vi "Ordena_Tags.vi"(0 "Tags_desorden":string[](array[string])) -> (1 "sorted array":i32[](array[numeric]), 2 "Array":string[](array[string]))   [LabVIEW 2015]
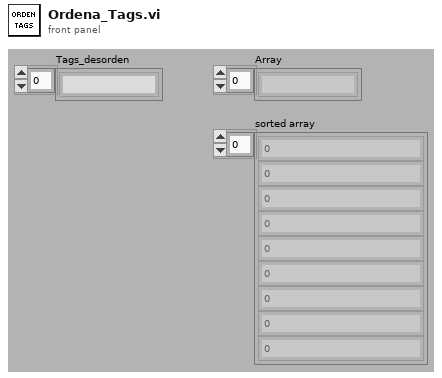
[diagram p1: front panel]
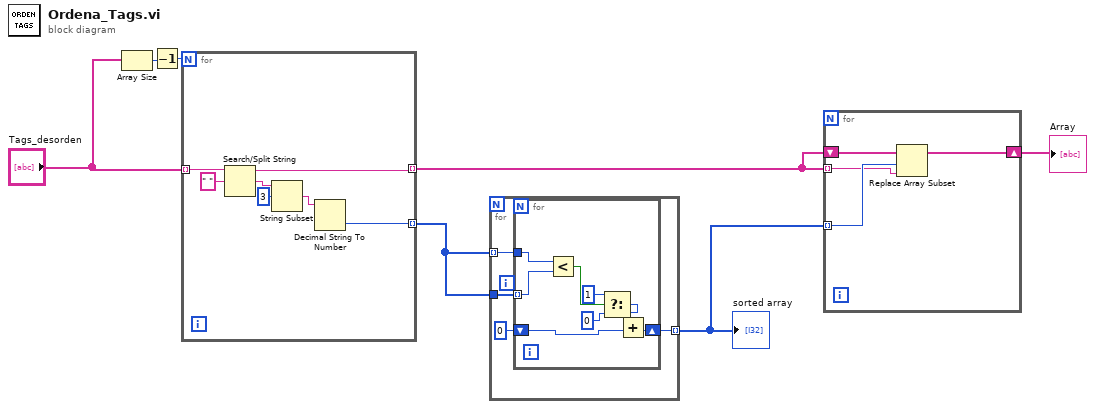
[diagram p0: block diagram]
diagram:
  n1 = Array Size(array="Tags_desorden") -> (size(s)=w1:i32)
  n2 = Decrement(x=w1) -> (x-1=w2:i32)
  n3 = for {
    N: w2 -> [_]
    tunnel: "Tags_desorden" -> [w14] mode=indexing
    tunnel: [w12] -> w5 mode=indexing
    tunnel: [w8] -> w3 mode=indexing
    n4 = Search/Split String(string=w14, search string/char (-)=" ") -> (substring before match=w12:string, match + rest of string=w11:string)  [unwired: 1 in, 1 out]
    n5 = String Subset(string=w11, offset (0)=3) -> (substring=w9:string)  [unwired: 1 in]
    n6 = Decimal String To Number(string=w9) -> (number=w8:i32)  [unwired: 2 in, 1 out]
  }
  n7 = for {
    tunnel: w3 -> [w18] mode=indexing
    tunnel: w3 -> [w17]
    tunnel: [w15] -> w4 mode=indexing
    n8 = for {
      tunnel: w18 -> [w26]
      tunnel: w17 -> [w25] mode=indexing
      shift-right: [w19] -> w15
      shift-left: 0 ("t") -> [w20]
      n9 = Less?(x=w26, y=w25) -> (x < y?=w24:bool)
      n10 = Select(t=1, s=w24, f=0 ("t")) -> (s? t:f=w21:i32)
      n11 = Add(x=w21, y=w20) -> (x+y=w19:i32)
    }
  }
  "sorted array" <- w4
  n12 = for {
    tunnel: w5 -> [w29] mode=indexing
    tunnel: w4 -> [w30] mode=indexing
    shift-right: [w27] -> w7
    shift-left: w5 -> [w28]
    n13 = Replace Array Subset(array=w28, new element=w29, index=w30) -> (w27:string[])
  }
  "Array" <- w7
